vi "Queuedmessage-ext.vi"() -> ()   [LabVIEW 2020]
panel:
  in  "Listbox":i32(listbox) caption="Select or double-click an item:"
  in  "Ring":u16(ring) caption="Change the value of the ring:" items=["Item 1", "Item 2", "Item 3"]
  in  "Button":bool caption="Press this button:"
  out "Last User Interface Event":string
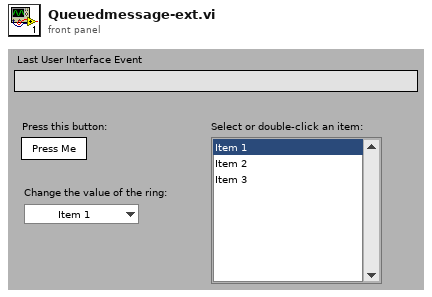
[diagram p1: front panel]
types:
  T1 = typedef "Queue RefNum" = refnum<k1>
  T2 = cluster{"last listbox value":i32, "last ring value":u16}
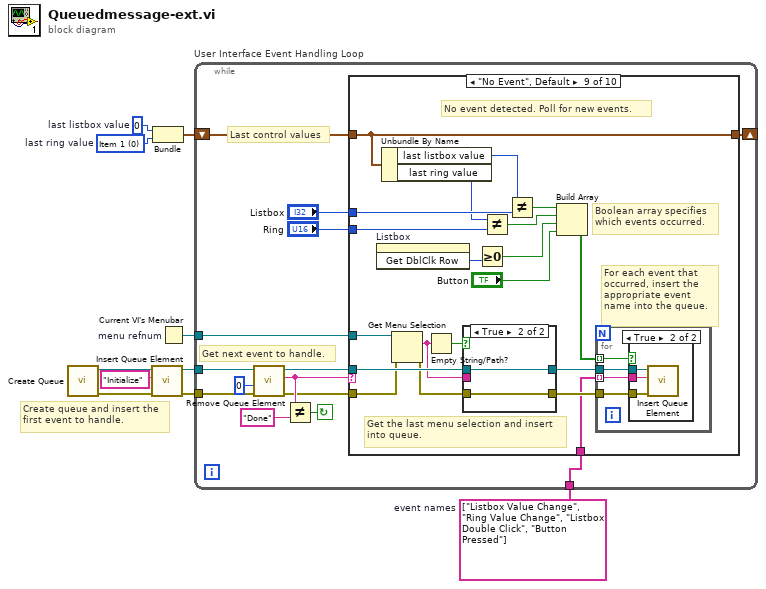
[diagram p0: block diagram]
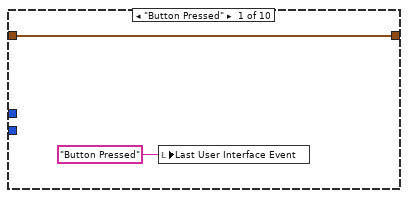
[diagram p2: hidden frame]
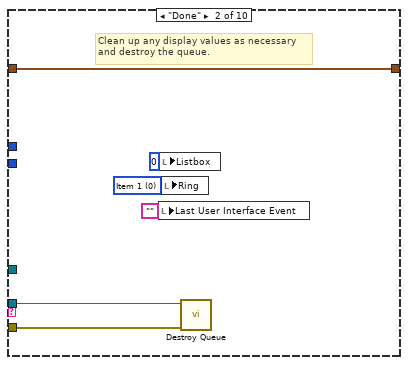
[diagram p3: hidden frame]
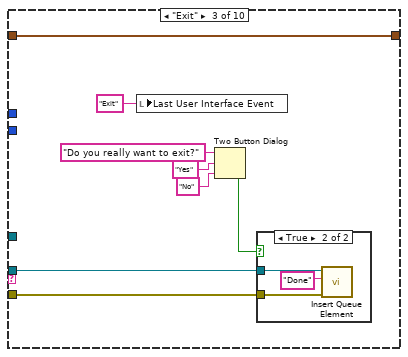
[diagram p4: hidden frame]
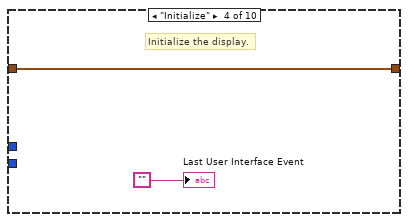
[diagram p6: hidden frame]
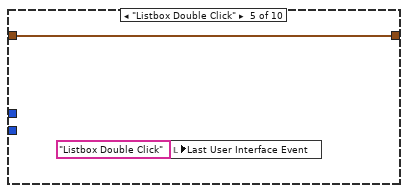
[diagram p7: hidden frame]
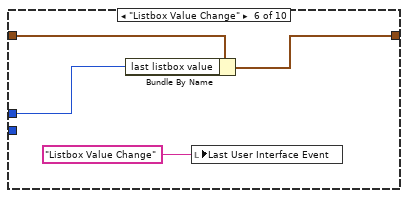
[diagram p8: hidden frame]
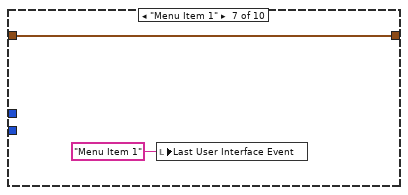
[diagram p9: hidden frame]
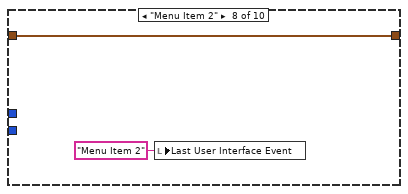
[diagram p10: hidden frame]
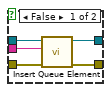
[diagram p11: hidden frame]
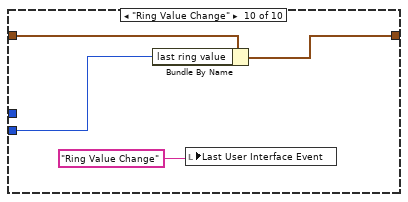
[diagram p13: hidden frame]
diagram:
  w7 = string[] ["Listbox Value Change", "Ring Value Change", "Listbox Double Click", "Button Pressed"]  # event names
  w8 = u16 0 items=["Item 1", "Item 2", "Item 3"]  # last ring value
  w9 = 0  # last listbox value
  # "Create queue and insert the\nfirst event to handle."
  n1 = call <vilib>:"Create Queue.vi"() -> ("error out"=w4:errorcluster, "queue out"=w5:T1)  [unwired: 4 in, 2 out]
  n2 = call <vilib>:"Insert Queue Element.vi"("error in (no error)"=w4, "queue element"="Initialize", "queue"=w5) -> ("error out"=w3:errorcluster, "queue out"=w6:T1)  [unwired: 2 in, 3 out]
  n3 = Bundle("last listbox value"=w9, "last ring value"=w8) -> (w10:T2)  [unwired: 1 out]
  n4 = Current VI's Menubar "menu refnum"() -> (w1:refnum<k9>)
  n5 = while "User Interface Event Handling Loop" {
    tunnel: w1 -> [w12]
    tunnel: w3 -> [w16]
    tunnel: w6 -> [w17]
    tunnel: w7 -> [w18]
    shift-left: w10 -> [w20]
    shift-right: [w19] -> _
    stop <- w23 continue-if-true
    # "Get next event to handle."
    # "Last control values"
    n6 = call <vilib>:"Remove Queue Element.vi"("error in (no error)"=w16, "ms timeout (-1)"=0, "queue"=w17) -> ("error out"=w13:errorcluster, "queue element"=w14:string, "queue out"=w15:T1)  [unwired: 1 in, 3 out]
    n7 = Not Equal?(x=w14, y="Done") -> (x != y?=w23:bool)
    n8 = case shown="\"No Event\", Default" w14 {
      tunnel: "Listbox" -> [_ _ _ _ _ w49 _ _ w73 _]
      tunnel: "Ring" -> [_ _ _ _ _ _ _ _ w71 w91]
      tunnel: w20 -> [w26 w32 w40 w45 w47 w51 w53 w55 w75 w93]
      tunnel: [w26 w32 w40 w45 w47 w50 w53 w55 w75 w92] -> w19
      tunnel: w15 -> [_ w28 w35 _ _ _ _ _ w65 _]
      tunnel: w18 -> [_ _ _ _ _ _ _ _ w57 _]
      tunnel: w13 -> [_ w27 w33 _ _ _ _ _ w64 _]
      tunnel: w12 -> [_ _ _ _ _ _ _ _ w61 _]
      frame "Button Pressed" {
        n9 = local write "Last User Interface Event"("Button Pressed" ("User Interface Event")) -> ()
      }
      frame "Done" {
        w30 = u16 0 items=["Item 1", "Item 2", "Item 3"] ("Ring")
        # "Clean up any display values as necessary\nand destroy the queue."
        n10 = local write "Last User Interface Event"("") -> ()
        n11 = local write "Listbox"(0 ("Listbox")) -> ()
        n12 = local write "Ring"(w30) -> ()
        n13 = call <vilib>:"Destroy Queue.vi"("error in (no error)"=w27, "queue"=w28) -> ()  [unwired: 6 out]
      }
      frame "Exit" {
        n14 = local write "Last User Interface Event"("Exit") -> ()
        n15 = Two Button Dialog(message="Do you really want to exit?", 1:"No" ("F button name (\"Cancel\")"), 2:"Yes" ("T button name (\"OK\")")) -> (T button?=w36:bool)
        n16 = case shown="True" w36 {
          tunnel: w35 -> [_ w42]
          tunnel: w33 -> [_ w43]
          frame False {
          }
          frame True {
            n17 = call <vilib>:"Insert Queue Element.vi"("error in (no error)"=w43, "queue element"="Done", "queue"=w42) -> ()  [unwired: 2 in, 5 out]
          }
        }
      }
      frame "Initialize" {
        # "Initialize the display."
        "Last User Interface Event" <- ""
      }
      frame "Listbox Double Click" {
        n18 = local write "Last User Interface Event"("Listbox Double Click" ("User Interface Event")) -> ()
      }
      frame "Listbox Value Change" {
        n19 = Bundle By Name(cluster=w51, "last listbox value"=w49) -> (w50:T2)
        n20 = local write "Last User Interface Event"("Listbox Value Change" ("User Interface Event")) -> ()
      }
      frame "Menu Item 1" {
        n21 = local write "Last User Interface Event"("Menu Item 1" ("User Interface Event")) -> ()
      }
      frame "Menu Item 2" {
        n22 = local write "Last User Interface Event"("Menu Item 2" ("User Interface Event")) -> ()
      }
      frame "No Event", Default {
        # "Get the last menu selection and insert\ninto queue."
        # "For each event that\noccurred, insert the\nappropriate event\nname into the queue."
        # "Boolean array specifies\nwhich events occurred."
        # "No event detected. Poll for new events."
        n23 = invoke on="Listbox" class="LstBox (strict)" method="Get DblClk Row"() -> ("Get DblClk Row"=w56:i32)  [unwired: 3 in, 2 out]
        n24 = Unbundle By Name(w75) -> ("last listbox value"=w74:i32, "last ring value"=w72:u16)
        n25 = Get Menu Selection(0:w61, 3:w64) -> (6:w59:string, 8:w63:errorcluster)  [unwired: 5 out]
        n26 = Empty String/Path?(string/path=w59) -> (empty?=w60:bool)
        n27 = case shown="True" w60 {
          tunnel: w65 -> [w77 w81]
          tunnel: w63 -> [w80 w82]
          tunnel: [w79 w82] -> w62
          tunnel: w59 -> [w78 _]
          tunnel: [w76 w81] -> w58
          frame False {
            n28 = call <vilib>:"Insert Queue Element.vi"("error in (no error)"=w80, "queue element"=w78, "queue"=w77) -> ("error out"=w79:errorcluster, "queue out"=w76:T1)  [unwired: 2 in, 3 out]
          }
          frame True {
          }
        }
        n29 = Greater Or Equal To 0?(x=w56) -> (x >= 0?=w68:bool)
        n30 = Not Equal?(x=w72, y=w71) -> (x != y?=w69:bool)
        n31 = Not Equal?(x=w74, y=w73) -> (x != y?=w70:bool)
        n32 = Build Array(w70, w69, w68, "Button") -> (w66:bool[])
        n33 = for {
          tunnel: w58 -> [w85]
          tunnel: w62 -> [w84]
          tunnel: w66 -> [w86] mode=indexing
          tunnel: w57 -> [w83] mode=indexing
          n34 = case shown="True" w86 {
            tunnel: w85 -> [_ w88]
            tunnel: w84 -> [_ w89]
            tunnel: w83 -> [_ w87]
            frame False {
            }
            frame True {
              n35 = call <vilib>:"Insert Queue Element.vi"("error in (no error)"=w89, "queue element"=w87, "queue"=w88) -> ()  [unwired: 2 in, 5 out]
            }
          }
        }
      }
      frame "Ring Value Change" {
        n36 = Bundle By Name(cluster=w93, "last ring value"=w91) -> (w92:T2)
        n37 = local write "Last User Interface Event"("Ring Value Change" ("Last User Interface Event")) -> ()
      }
    }
  }
